vi "NodeLookup.vi"(4 "String":string, 5 "Boolean":bool=TRUE) -> (1 "Numeric":i32)   [LabVIEW 2011]
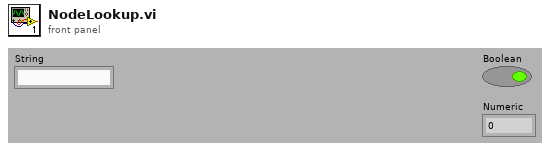
[diagram p1: front panel]
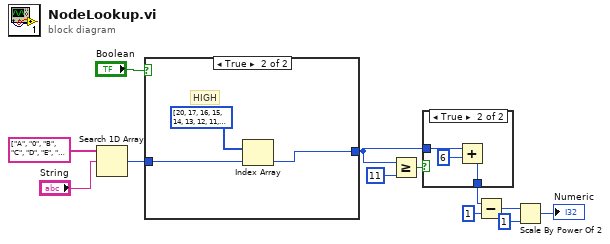
[diagram p0: block diagram]
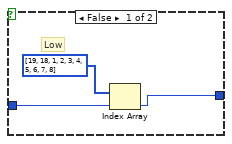
[diagram p3: hidden frame]
diagram:
  n1 = Search 1D Array(1D array=string[] ["A", "0", "B", "C", "D", "E", "F", "G", "H", "I"], element="String") -> (index of element=w9:i32)  [unwired: 1 in]
  n2 = case shown="True" "Boolean" {
    tunnel: w9 -> [w15 w18]
    tunnel: [w14 w17] -> w1
    frame False {
      # "Low"
      n3 = Index Array(array=i32[] [19, 18, 1, 2, 3, 4, 5, 6, 7, 8], index=w15) -> (element=w14:i32)
    }
    frame True {
      # "HIGH"
      n4 = Index Array(array=i32[] [20, 17, 16, 15, 14, 13, 12, 11, 10, 9], index=w18) -> (element=w17:i32)
    }
  }
  n5 = Greater Or Equal?(x=w1, y=11) -> (x >= y?=w5:bool)
  n6 = case shown="True" w5 {
    tunnel: w1 -> [w19 w22]
    tunnel: [w19 w20] -> w8
    frame False {
    }
    frame True {
      n7 = Add(x=w22, y=6) -> (x+y=w20:i32)
    }
  }
  n8 = Subtract(x=w8, y=1) -> (x-y=w3:i32)
  n9 = Scale By Power Of 2(n=w3, x=1) -> (x*2^n=→"Numeric":i32)
